vi "GPS Coordinates to distance.vi"(10 "GPS Co-ordinate 2":T1 {"Longitude" format="%#_14g"; "Latitude" format="%#_14g"}, 11 "GPS Co-ordinate 1":T1 {"Longitude" format="%#_14g"; "Latitude" format="%#_14g"}) -> (3 "Distance":dbl)   [LabVIEW 2009]
uses:
  TypeDefs/Sensor TypeDefs/GPS Data.ctl
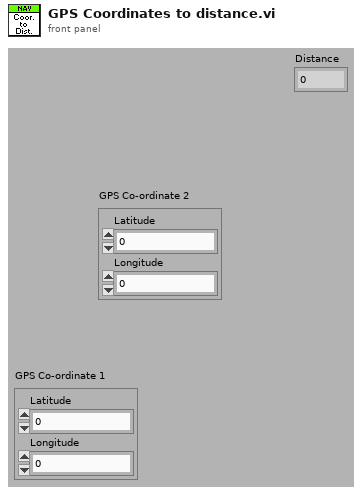
[diagram p1: front panel]
types:
  T1 = typedef "GPS Data.ctl" = cluster{"Latitude":dbl, "Longitude":dbl}
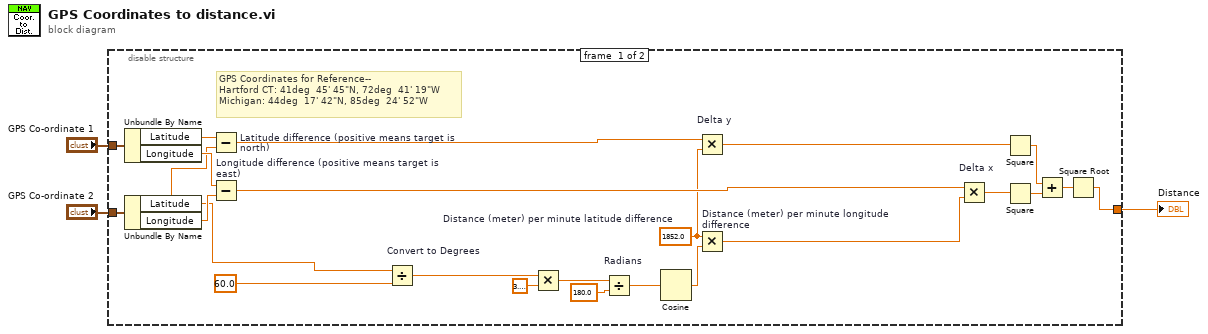
[diagram p0: block diagram]
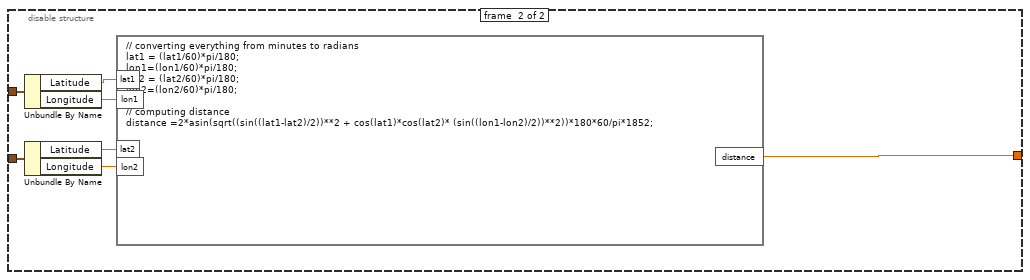
[diagram p2: hidden frame]
diagram:
  n1 = disable-structure shown="Enabled" {
    disable-tunnel: [w19 w27] -> w3
    disable-tunnel: "GPS Co-ordinate 2" -> [w16 w30]
    disable-tunnel: "GPS Co-ordinate 1" -> [w15 w33]
    frame #0 {
      w21 = 1852.0  # Distance (meter) per minute latitude difference
      # "GPS Coordinates for Reference--\nHartford CT: 41deg  45' 45\"N, 72deg  41' 19\"W\nMichigan: 44deg  17' 42\"N, 85deg  24' 52\"W"
      n2 = Unbundle By Name(w15) -> ("Latitude"=w8:dbl, "Longitude"=w7:dbl)
      n3 = Unbundle By Name(w16) -> ("Latitude"=w4:dbl, "Longitude"=w6:dbl)
      n4 = Subtract "Latitude difference (positive means target is north)"(x=w8, y=w4) -> (x-y=w23:dbl)
      n5 = Subtract "Longitude difference (positive means target is east)"(x=w7, y=w6) -> (x-y=w22:dbl)
      n6 = Divide "Convert to Degrees"(x=w4, y=60.0) -> (x/y=w12:dbl)
      n7 = Multiply(x=w12, y=3.141592653589793) -> (x*y=w11:dbl)
      n8 = Divide "Radians"(x=w11, y=180.0) -> (x/y=w9:dbl)
      n9 = Cosine(x=w9) -> (cos(x)=w5:dbl)
      n10 = Multiply "Delta y"(x=w23, y=w21) -> (x*y=w17:dbl)
      n11 = Multiply "Distance (meter) per minute longitude difference"(x=w21, y=w5) -> (x*y=w20:dbl)
      n12 = Multiply "Delta x"(x=w22, y=w20) -> (x*y=w18:dbl)
      n13 = Square(x=w17) -> (x^2=w26:dbl)
      n14 = Square(x=w18) -> (x^2=w25:dbl)
      n15 = Add(x=w26, y=w25) -> (x+y=w24:dbl)
      n16 = Square Root(x=w24) -> (sqrt(x)=w19:dbl)
    }
    frame #1 {
      n17 = Unbundle By Name(w33) -> ("Latitude"=w32:dbl, "Longitude"=w31:dbl)
      n18 = Unbundle By Name(w30) -> ("Latitude"=w29:dbl, "Longitude"=w28:dbl)
      n19 = formula code="// converting everything from minutes to radians\nlat1 = (lat1/60)*pi/180;\nlon1=(lon1/60)*pi/180;\nlat2 = (lat2/60)*pi/180;\nlon2=(lon2/60)*pi/180;\n\n// computing distance\ndistance =2*asin(sqrt((sin((lat1-lat2)/2))**2 + cos(lat1)*cos(lat2)* (sin((lon1-lon2)/2))**2))*180*60/pi*1852;"("lon1"=w31, "lat1"=w32, "lat2"=w29, "lon2"=w28) -> ("distance"=w27:dbl)
    }
  }
  "Distance" <- w3
